vi "diagram_disable_structure.vi"() -> ()   [LabVIEW 2019]
panel:
  out "output 6":bool
  in  "a 6":dbl
  out "output 5":bool
  in  "a 5":dbl
  out "output 4":bool
  in  "a 4":dbl
  out "output 3":bool
  in  "a 3":dbl
  out "output 2":bool
  in  "a 2":dbl
  out "output":bool
  in  "a":dbl
  # "DIAGRAM DISABLE STRUCTURE AND COMPARISON FUNCTION"
  # "Equal to / not equal to comparison"
  # "greater than/less than"
  # "LESS THAN OR EUAL TO / GREATER THAN OR EQUAL TO"
  # "EQUAL TO ZERO / NOT EQUAL TO ZERO"
  # "GREATER THAN  ZERO / LESS THAN ZERO"
  # "GREATER THAN OR EQUAL TO ZERO / LESS THAN OR EQUAL TO ZERO"
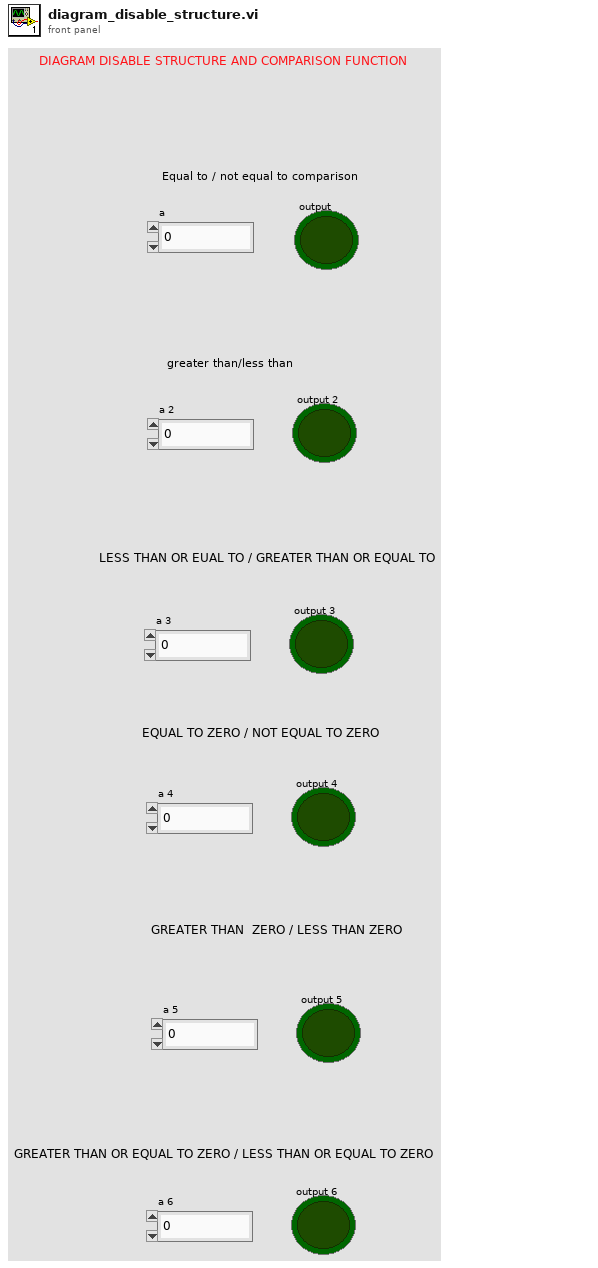
[diagram p1: front panel]
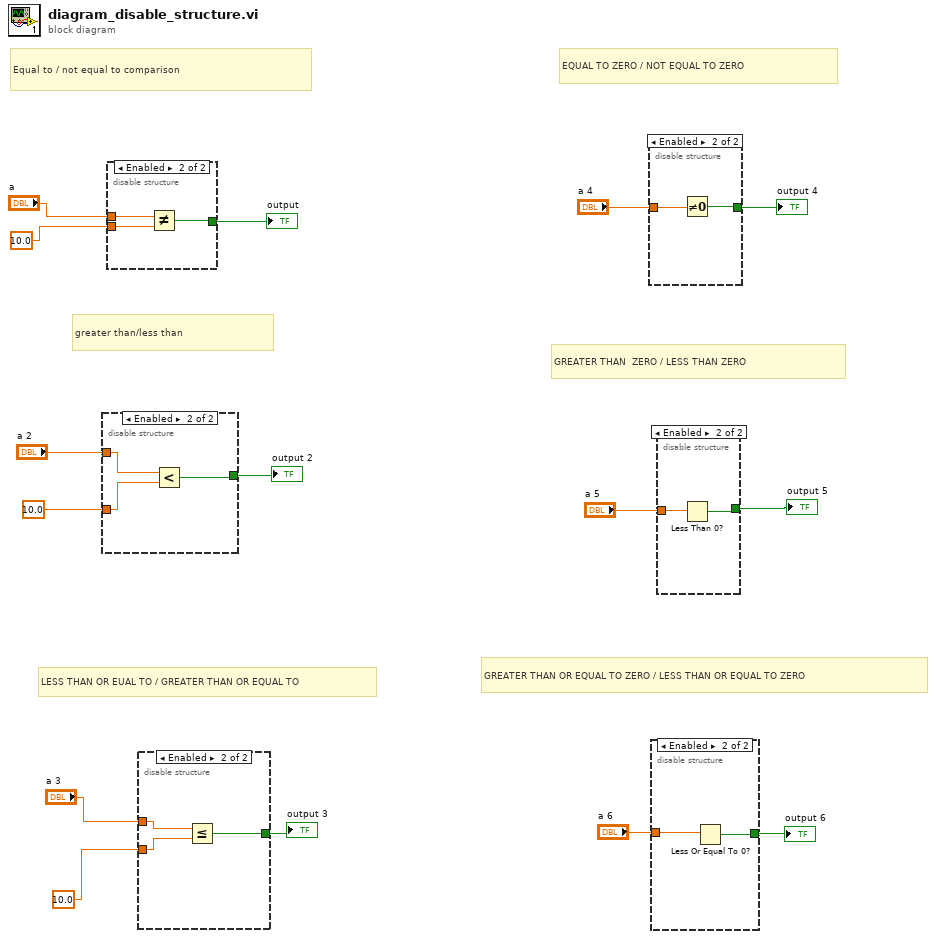
[diagram p0: block diagram]
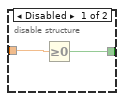
[diagram p2: hidden frame]
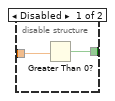
[diagram p3: hidden frame]
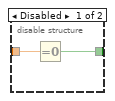
[diagram p4: hidden frame]
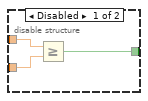
[diagram p5: hidden frame]
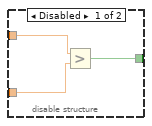
[diagram p6: hidden frame]
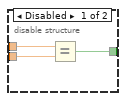
[diagram p7: hidden frame]
diagram:
  # "GREATER THAN OR EQUAL TO ZERO / LESS THAN OR EQUAL TO ZERO"
  # "GREATER THAN  ZERO / LESS THAN ZERO"
  # "EQUAL TO ZERO / NOT EQUAL TO ZERO"
  # "LESS THAN OR EUAL TO / GREATER THAN OR EQUAL TO"
  # "greater than/less than"
  # "Equal to / not equal to comparison"
  n1 = disable-structure shown="Enabled" {
    disable-tunnel: "a 2" -> [w18 w21]
    disable-tunnel: 10.0 ("y") -> [w17 w20]
    disable-tunnel: [w16 w19] -> w10
    frame Disabled {
      n2 = Greater?(x=w18, y=w17) -> (0:w16:bool)
    }
    frame Enabled {
      n3 = Less?(x=w21, y=w20) -> (x < y?=w19:bool)
    }
  }
  "output 2" <- w10
  n4 = disable-structure shown="Enabled" {
    disable-tunnel: [w24 w25] -> w15
    disable-tunnel: "a" -> [w23 w27]
    disable-tunnel: 10.0 ("y") -> [w22 w26]
    frame Disabled {
      n5 = Equal?(x=w23, y=w22) -> (x = y?=w24:bool)
    }
    frame Enabled {
      n6 = Not Equal?(x=w27, y=w26) -> (x != y?=w25:bool)
    }
  }
  "output" <- w15
  n7 = disable-structure shown="Enabled" {
    disable-tunnel: "a 3" -> [w30 w33]
    disable-tunnel: 10.0 ("y") -> [w29 w32]
    disable-tunnel: [w28 w31] -> w7
    frame Disabled {
      n8 = Greater Or Equal?(x=w30, y=w29) -> (x >= y?=w28:bool)
    }
    frame Enabled {
      n9 = Less Or Equal?(x=w33, y=w32) -> (x <= y?=w31:bool)
    }
  }
  "output 3" <- w7
  n10 = disable-structure shown="Enabled" {
    disable-tunnel: "a 4" -> [w35 w37]
    disable-tunnel: [w34 w36] -> w5
    frame Disabled {
      n11 = Equal To 0?(x=w35) -> (x = 0?=w34:bool)
    }
    frame Enabled {
      n12 = Not Equal To 0?(x=w37) -> (x != 0?=w36:bool)
    }
  }
  "output 4" <- w5
  n13 = disable-structure shown="Enabled" {
    disable-tunnel: "a 6" -> [w39 w41]
    disable-tunnel: [w38 w40] -> w1
    frame Disabled {
      n14 = Greater Or Equal To 0?(x=w39) -> (x >= 0?=w38:bool)
    }
    frame Enabled {
      n15 = Less Or Equal To 0?(x=w41) -> (x <= 0?=w40:bool)
    }
  }
  "output 6" <- w1
  n16 = disable-structure shown="Enabled" {
    disable-tunnel: "a 5" -> [w43 w45]
    disable-tunnel: [w42 w44] -> w3
    frame Disabled {
      n17 = Greater Than 0?(x=w43) -> (x > 0?=w42:bool)
    }
    frame Enabled {
      n18 = Less Than 0?(x=w45) -> (x < 0?=w44:bool)
    }
  }
  "output 5" <- w3
